vi "Change Control Mode.vi"(6 "Control Mode":u8(ring) items=["Velocity"=2, "Torque"=1], 7 "timeout (1s)":dbl=1.0 min=0.0, 8 "error in (no error)":errorcluster, 11 "SDO object in":refnum<k20>) -> (0 "error out":errorcluster, 1 "completion code 2":u32, 2 "completion code 1":u32, 3 "SDO object out":refnum<k20>)   [LabVIEW 2016]
uses:
  Set mode of operation.vi
  Set control mode.vi
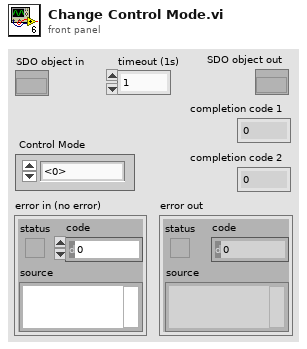
[diagram p1: front panel]
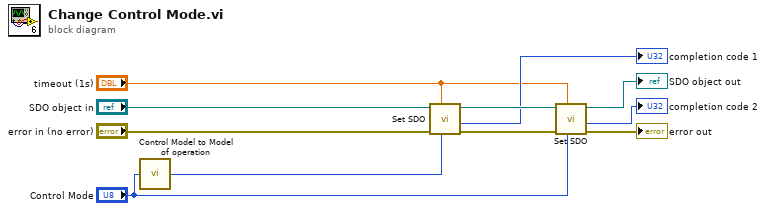
[diagram p0: block diagram]
diagram:
  n1 = call "Control Model to Model of operation.vi"("Control Mode"="Control Mode") -> ("Mode of operation"=w9:i8)
  n2 = call-poly "Set SDO.vi"("Mode of operation"=w9, "timeout (1s)"="timeout (1s)", "error in (no error)"="error in (no error)", "SDO object in"="SDO object in") -> ("error out"=w10:errorcluster, "completion code"=→"completion code 1":u32, "SDO object out"=w11:refnum<k20>)  [unwired: 5 in]
  n3 = call-poly "Set SDO.vi"("Control Mode"="Control Mode", "timeout (1s)"="timeout (1s)", "error in (no error)"=w10, "SDO object in"=w11) -> ("error out"=→"error out":errorcluster, "completion code"=→"completion code 2":u32, "SDO object out"=→"SDO object out":refnum<k20>)  [unwired: 5 in]
